vi "New Queue Sink.vi"(8 "error in (no error)":errorcluster, 11 "Queue Name":string) -> (0 "error out":errorcluster, 3 "Queue Sink out":refnum<class "Queue Sink.lvclass">)   [LabVIEW 2020, in "LV Log.lvlib" / "Queue Sink.lvclass"]
uses:
  Queue Sink.lvclass
  Queue Sink.lvclass/Queue Sink.ctl
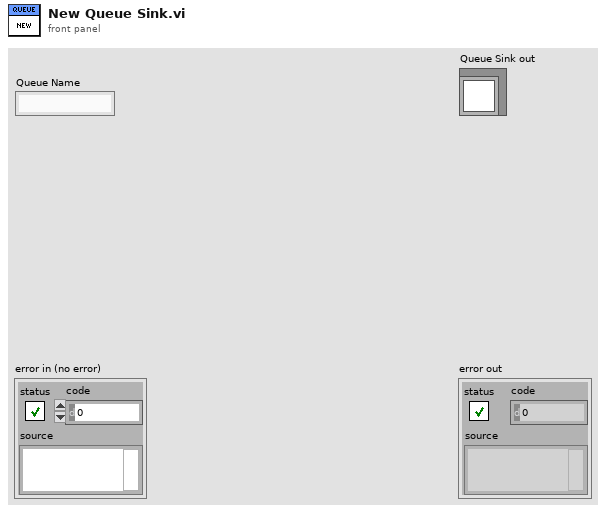
[diagram p1: front panel]
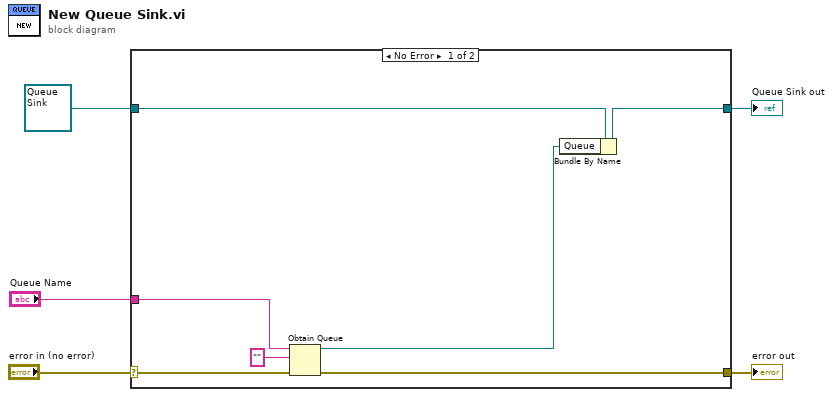
[diagram p0: block diagram]
diagram:
  n1 = case shown="No Error" "error in (no error)" {
    selector: "error in (no error)" -> [w12 w14]
    tunnel: [w11 w14] -> w4
    tunnel: [w8 w13] -> w2
    tunnel: refnum<class "Queue Sink.lvclass"> refnum ("Queue Sink in") -> [w9 w13]
    tunnel: "Queue Name" -> [w6 _]
    frame No Error {
      n2 = Obtain Queue(name (unnamed)=w6, element data type="", error in (no error)=w12) -> (queue out=w7:refnum<queue>, error out=w11:errorcluster)  [unwired: 2 in, 1 out]
      n3 = Bundle By Name(cluster=w9, "Queue"=w7) -> (w8:refnum<class "Queue Sink.lvclass">)
    }
    frame Error {
    }
  }
  "error out" <- w4
  "Queue Sink out" <- w2
